vi "UsrProfiles-Copy profile path.vi"   [LabVIEW 2020]
uses:
  Globals/gl_UsrProfiles globals.vi
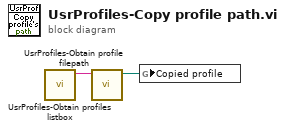
[diagram p0: block diagram]
diagram:
  n1 = call "UsrProfiles-Obtain profiles listbox.vi"() -> ("Selected profile's name"=w2:string)  [unwired: 8 in, 3 out]
  n2 = call "UsrProfiles-Obtain profile filepath.vi"("Profile name"=w2) -> ("Profile filepath"=w1:path)  [unwired: 9 in, 1 out]
  n3 = global write "gl_UsrProfiles globals.vi" "Copied profile"(w1) -> ()
